vi "Retrieve_latest_PAQ_data.vi"(8 "error in (no error)":errorcluster, 10 "FetchLatestDefinition":T2, 11 "DBAL-BIN in":refnum<class "DBAL-BIN.lvclass">) -> (0 "error out":errorcluster, 2 "BinHistData":T1, 3 "DBAL-BIN out":refnum<class "DBAL-BIN.lvclass">)   [LabVIEW 2020, in "DBAL-BIN.lvclass"]
uses:
  DBAL-BIN.lvclass
  controls/DBAL_FetchLatestFrom.ctl
  controls/BIN/BINdata.ctl
  DBAL-BIN.lvclass/DBAL-BIN.ctl
  Common/controls/Global-test.vi
panel:
  out "String":string
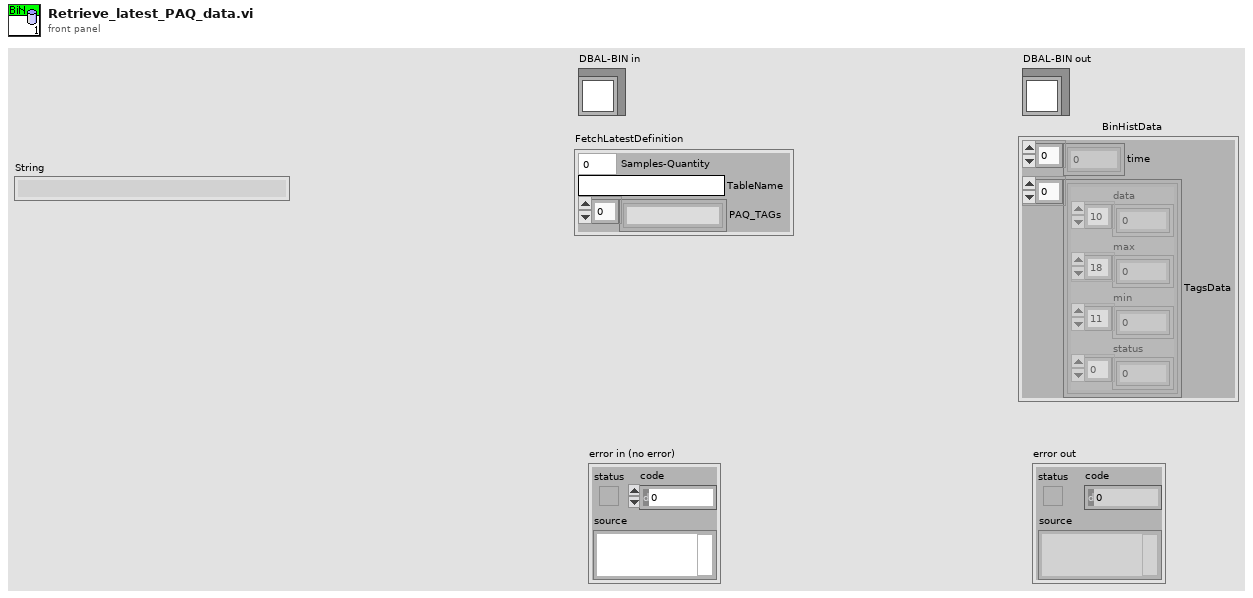
[diagram p1: front panel]
types:
  T1 = typedef "DBAL-BIN.lvclass/BINdata.ctl" = cluster{"time":dbl[], "TagsData":cluster{"data":dbl[], "max":dbl[], "min":dbl[], "status":u32[]}[]}
  T2 = typedef "DBAL_FetchLatestFrom.ctl" = cluster{"Samples-Quantity":i32, "TableName":string, "PAQ_TAGs":string[]}
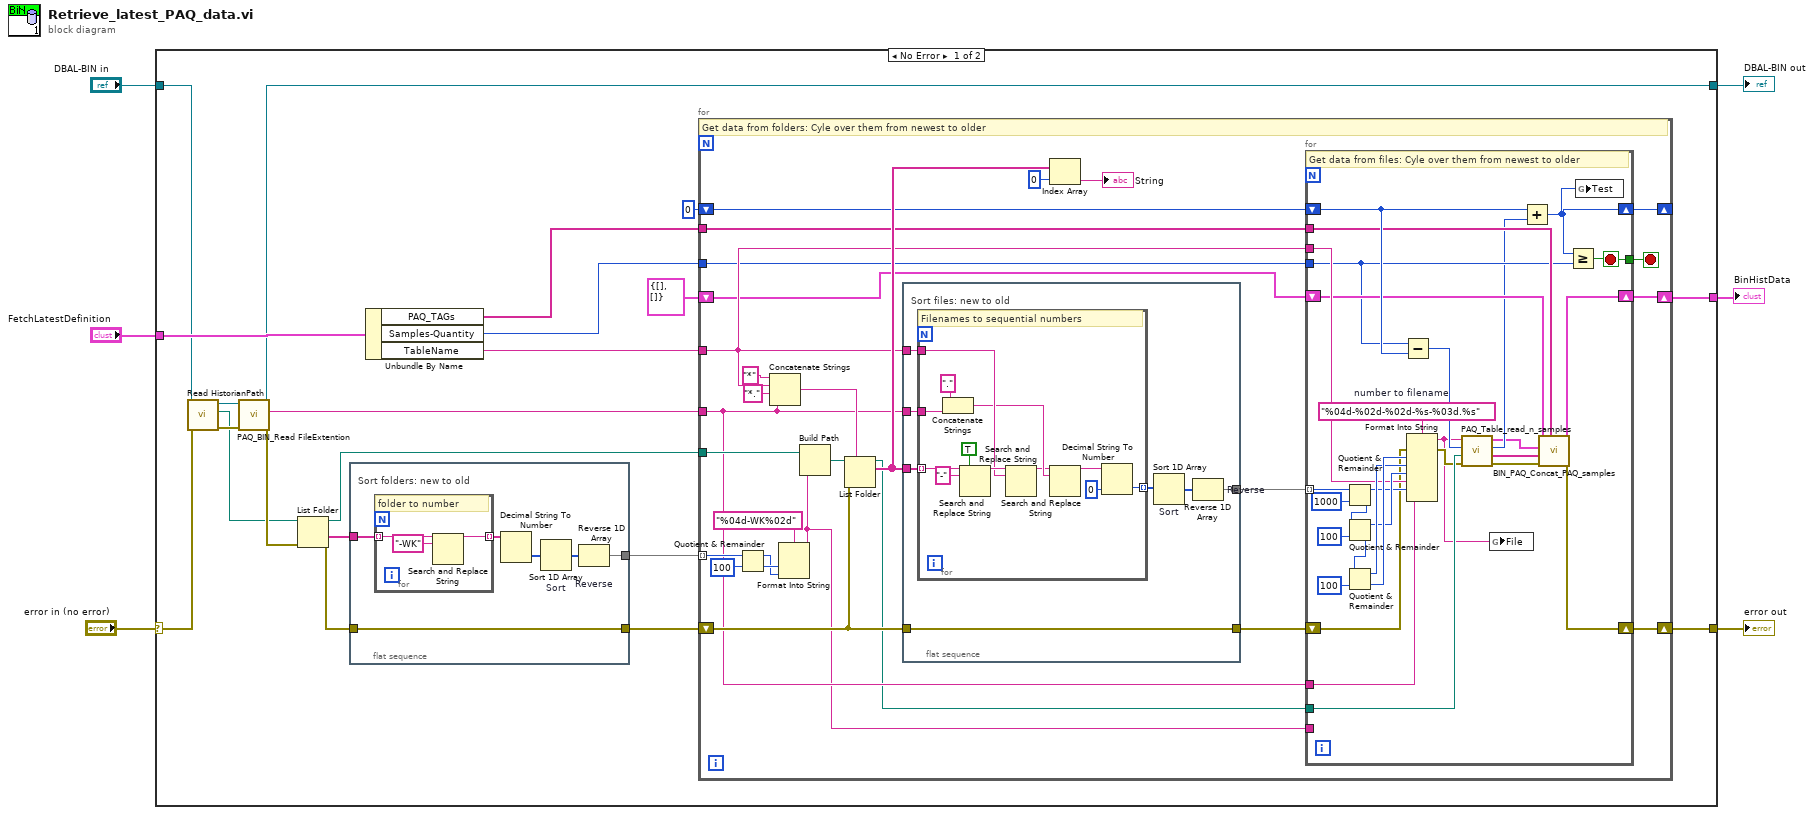
[diagram p0: block diagram]
diagram:
  n1 = case shown="No Error" "error in (no error)" {
    selector: "error in (no error)" -> [w15 w114]
    tunnel: [w21 w114] -> w5
    tunnel: "DBAL-BIN in" -> [w16 w115]
    tunnel: [w10 w115] -> w3
    tunnel: "FetchLatestDefinition" -> [w27 _]
    tunnel: [w7 _] -> w1
    frame No Error {
      n2 = call "Read HistorianPath.vi"("error in (no error)"=w15, "DBAL-BIN in"=w16) -> ("error out"=w14:errorcluster, "HistorianPath"=w13:path, "DBAL-BIN out"=w17:refnum<class "DBAL-BIN.lvclass">)  [unwired: 7 in]
      n3 = call "PAQ_BIN_Read FileExtention.vi"("error in (no error)"=w14, "DBAL-BIN in"=w17) -> ("error out"=w18:errorcluster, "FileExtention"=w19:string, "DBAL-BIN out"=w10:refnum<class "DBAL-BIN.lvclass">)  [unwired: 7 in]
      n4 = List Folder(path=w13, error in=w18) -> (path out=w26:path, folder names=w22:string[], error out=w23:errorcluster)  [unwired: 2 in, 1 out]
      n5 = flat-sequence {
        tunnel: w22 -> [w110]
        tunnel: [w105] -> w25
        tunnel: w23 -> [w107]
        tunnel: [w107] -> w24
        frame #0 {
          # "Sort folders: new to old"
          n6 = for {
            tunnel: w110 -> [w113] mode=indexing
            tunnel: [w111] -> w109 mode=indexing
            # "folder to number"
            n7 = Search and Replace String(input string=w113, search string="-WK") -> (result string=w111:string)  [unwired: 6 in, 3 out]
          }
          n8 = Decimal String To Number ("to num")(string=w109) -> (number=w108:i32[])  [unwired: 2 in, 1 out]
          n9 = Sort 1D Array "Sort"(array=w108) -> (sorted array=w106:i32[])
          n10 = Reverse 1D Array "Reverse"(array=w106) -> (reversed array=w105:i32[])
        }
      }
      n11 = Unbundle By Name(w27) -> ("PAQ_TAGs"=w9:string[], "Samples-Quantity"=w12:i32, "TableName"=w20:string)
      n12 = for {
        shift-right: [w36] -> w21
        shift-left: w24 -> [w45]
        tunnel: w25 -> [w55] mode=indexing
        tunnel: w19 -> [w39]
        tunnel: w26 -> [w50]
        tunnel: w20 -> [w40]
        tunnel: w12 -> [w35]
        shift-right: [w33] -> _
        shift-left: 0 ("Fetched samples") -> [w34]
        tunnel: w9 -> [w32]
        shift-right: [w31] -> w7
        shift-left: T1 {"time"=[], "TagsData"=[]} ("BinHistData") -> [w30]
        stop <- w29 stop-if-true
        # "Get data from folders: Cyle over them from newest to older"
        n13 = Quotient & Remainder(x=w55, y=100) -> (x-y*floor(x/y)=w51:i32, floor(x/y)=w52:i32)
        n14 = Concatenate Strings("*", w40, "*.", w39) -> (w46:string)
        n15 = Format Into String(format string="%04d-WK%02d", w52, w51) -> (resulting string=w28:string)  [unwired: 2 in, 1 out]
        n16 = Build Path(base path=w50, name or relative path=w28) -> (appended path=w49:path)
        n17 = List Folder(path=w49, pattern=w46, error in=w45) -> (path out=w38:path, filenames=w43:string[])  [unwired: 1 in, 2 out]
        n18 = flat-sequence {
          tunnel: w43 -> [w92]
          tunnel: w40 -> [w91]
          tunnel: w39 -> [w90]
          tunnel: [w87] -> w44
          tunnel: w45 -> [w86]
          tunnel: [w86] -> w37
          frame #0 {
            # "Sort files: new to old"
            n19 = for {
              tunnel: w92 -> [w93] mode=indexing
              tunnel: w91 -> [w101]
              tunnel: w90 -> [w100]
              tunnel: [w95] -> w88 mode=indexing
              # "Filenames to sequential numbers"
              n20 = Concatenate Strings("." ("string"), w100) -> (w99:string)
              n21 = Search and Replace String(replace all?=TRUE ("replace all? (F)"), input string=w93, search string="-") -> (result string=w102:string)  [unwired: 5 in, 3 out]
              n22 = Search and Replace String(input string=w102, search string=w101) -> (result string=w98:string)  [unwired: 6 in, 3 out]
              n23 = Search and Replace String(input string=w98, search string=w99) -> (result string=w96:string)  [unwired: 6 in, 3 out]
              n24 = Decimal String To Number(string=w96, default (0L)=u64 0 ("default (0 I32)")) -> (number=w95:u64)  [unwired: 1 in, 1 out]
            }
            n25 = Sort 1D Array "Sort"(array=w88) -> (sorted array=w89:u64[])
            n26 = Reverse 1D Array "Reverse"(array=w89) -> (reversed array=w87:u64[])
          }
        }
        n27 = Index Array(array=w43, index=0) -> (element=→"String":string)
        n28 = for {
          tunnel: w44 -> [w84] mode=indexing
          tunnel: w40 -> [w75]
          tunnel: w39 -> [w73]
          tunnel: w38 -> [w71]
          shift-right: [w64] -> w36
          shift-left: w37 -> [w72]
          tunnel: w35 -> [w61]
          shift-right: [w57] -> w33
          shift-left: w34 -> [w68]
          tunnel: w32 -> [w62]
          shift-right: [w66] -> w31
          shift-left: w30 -> [w67]
          tunnel: [w60] -> w29
          tunnel: w28 -> [_]
          stop <- w60 stop-if-true
          w79 = "%04d-%02d-%02d-%s-%03d.%s"  # number to filename
          # "Get data from files: Cyle over them from newest to older"
          n29 = Quotient & Remainder(x=w84, y=u64 1000) -> (x-y*floor(x/y)=w74:u64, floor(x/y)=w82:u64)
          n30 = Quotient & Remainder(x=w82, y=u64 100) -> (x-y*floor(x/y)=w76:u64, floor(x/y)=w80:u64)
          n31 = Quotient & Remainder(x=w80, y=u64 100) -> (x-y*floor(x/y)=w77:u64, floor(x/y)=w78:u64)
          n32 = Subtract(x=w61, y=w68) -> (x-y=w69:i32)
          n33 = Format Into String(format string=w79, error in=w72, w78, w77, w76, w75, w74, w73) -> (resulting string=w56:string, error out=w70:errorcluster)  [unwired: 1 in]
          n34 = call "PAQ_Table_read_n_samples.vi"("error in (no error)"=w70, "Sub Path"=w71, "Required samples"=w69, "Table Filename"=w56) -> ("error out"=w65:errorcluster, "TAGs"=w63:string[], "Fetched samples"=w59:i32, "value"=w58:T1)  [unwired: 4 in]
          n35 = global write "Global-test.vi" "File"(w56) -> ()
          n36 = Add(x=w68, y=w59) -> (x+y=w57:i32)
          n37 = call "BIN_PAQ_Concat_PAQ_samples.vi"("Memory TAGs"=w62, "error in (no error)"=w65, "Added samples TAGs"=w63, "PAQ Samples to ADD"=w58, "PAQ Samples IN"=w67) -> ("error out"=w64:errorcluster, "PAQ Samples OUT"=w66:T1)  [unwired: 5 in]
          n38 = Greater Or Equal?(x=w57, y=w61) -> (x >= y?=w60:bool)
          n39 = global write "Global-test.vi" "Test"(w57) -> ()
        }
      }
    }
    frame Error {
    }
  }
  "error out" <- w5
  "DBAL-BIN out" <- w3
  "BinHistData" <- w1
